vi "TiePie.Lst.LstRemoveDevice.vi"(8 "error in (no error)":errorcluster) -> (0 "error out":errorcluster, 11 "deSerialNumber":u32)   [LabVIEW 2014, in "LVTiePie.lvlib"]
uses:
  LVTiePie.lvlib
  bin/libtiepie.dll
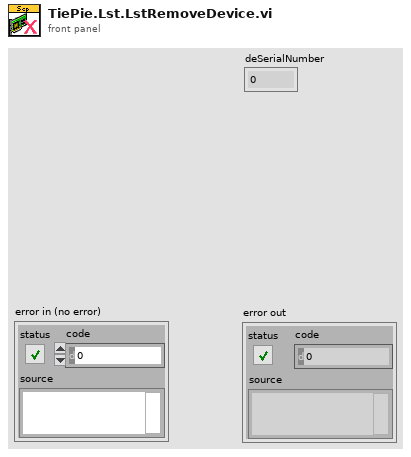
[diagram p1: front panel]
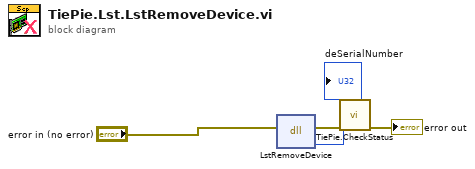
[diagram p0: block diagram]
diagram:
  n1 = dll-call lib="C:/Users/mbirski/Desktop/PAN/LabVEW/Tie Pie/bin/libtiepie.dll" fn="LstRemoveDevice"(error in="error in (no error)") -> (error out=w3:errorcluster, "deSerialNumber"=→"deSerialNumber":u32)  [unwired: 4 in, 1 out]
  n2 = call "TiePie.CheckStatus.vi"("error in (no error)"=w3) -> ("error out"=→"error out":errorcluster)  [unwired: 10 in]
